vi "Init Serial Port.vi"(8 "error in (no error)":errorcluster, 9 "Input\nbuffer size":u32=4096, 10 "baud rate":u32=9600, 11 "VISA Refnum in":refnum<visa-resource-name>) -> (0 "error out":errorcluster, 3 "VISA Refnum out":refnum<visa-resource-name>)   [LabVIEW 2013]
doc: "opens a serial port (on the RIO or a standard computer) and sets up the buffers so they actually work.\n-Jason"
uses:
  <vilib>/Instr/_visa.llb/VISA Configure Serial Port (Instr).vi
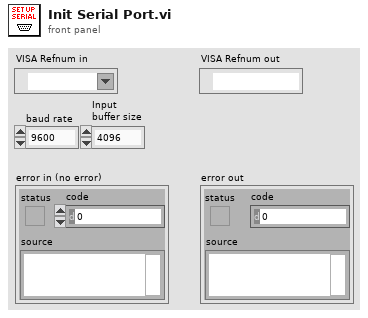
[diagram p1: front panel]
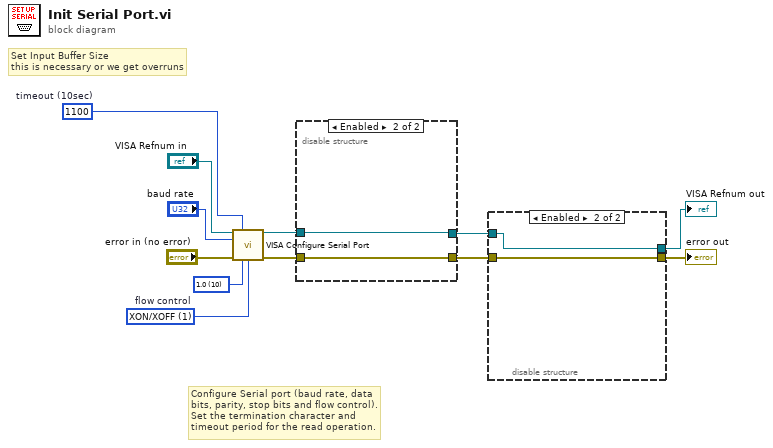
[diagram p0: block diagram]
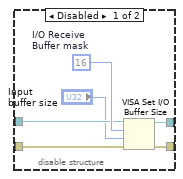
[diagram p2: hidden frame]
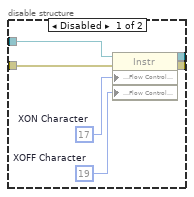
[diagram p3: hidden frame]
diagram:
  w2 = u16 10 items=["1.0"=10, "1.5"=15, "2.0"=20] ("stop bits (10: 1 bit)")
  w8 = u32 1100  # timeout (10sec)
  w4 = u16 1 items=["None"=0, "XON/XOFF"=1, "RTS/CTS"=2, "DTR/DSR"=4]  # flow control
  # "Set Input Buffer Size\nthis is necessary or we get overruns"
  # "Configure Serial port (baud rate, data\nbits, parity, stop bits and flow control).\nSet the termination character and\ntimeout period for the read operation."
  n1 = call-poly "VISA Configure Serial Port"("VISA resource name"="VISA Refnum in", "timeout (10sec)"=w8, "baud rate (9600)"="baud rate", "error in (no error)"="error in (no error)", "stop bits (10: 1 bit)"=w2, "flow control (0:none)"=w4) -> ("VISA resource name out"=w6:refnum<visa-resource-name>, "error out"=w7:errorcluster)  [unwired: 8 in]
  n2 = disable-structure shown="Enabled" {
    disable-tunnel: w7 -> [w17 w19]
    disable-tunnel: w6 -> [w16 w20]
    disable-tunnel: [w15 w20] -> w5
    disable-tunnel: [w13 w19] -> w1
    frame Disabled {
      w18 = u16 16  # I/O Receive Buffer mask
      n3 = VISA Set I/O Buffer Size(VISA resource name=w16, mask (16)=w18, size (4096)="Input\nbuffer size", error in (no error)=w17) -> (VISA resource name out=w15:refnum<visa-resource-name>, error out=w13:errorcluster)
    }
    frame Enabled {
    }
  }
  n4 = disable-structure shown="Enabled" {
    disable-tunnel: [w26 w27] -> w12
    disable-tunnel: [w25 w28] -> w11
    disable-tunnel: w5 -> [w21 w28]
    disable-tunnel: w1 -> [w22 w27]
    frame Disabled {
      w24 = u8 19  # XOFF Character
      w23 = u8 17  # XON Character
      n5 = property class="Instr"(reference=w21, error in=w22, "Serial Settings:Flow Control XON Character"=w23, "Serial Settings:Flow Control XOFF Character"=w24) -> (reference out=w25:refnum<visa-resource-name>, error out=w26:errorcluster)
    }
    frame Enabled {
    }
  }
  "error out" <- w12
  "VISA Refnum out" <- w11
